vi "SQL_DB.vi"(3 "column information":T2[](array[typedef]), 4 "Column Names":T1=["Barcode", "[Date&Time]", "[User Name]", "Shift", "Model", "Variant", "[Test Name]", "[Test Type]", "[Excepted Value]", "HL", "LL", "[Obtained Value]", "Result", "[Cycle Time]"], 5 "datatype":string[][](array[string]), 6 "Table Name":string, 7 "CTRL":T4=enum."Open Connections", 8 "error in (no error)":errorcluster, 9 "SQL query":string, 10 "data to Update":variant, 11 "Connection Info":string="Provider=SQLNCLI11;Server=ADMIN-PC;Database=mmk;Trusted_Connection=yes;") -> (0 "error in (no error) 2":errorcluster, 1 "Data out 2":string[][](array[string]), 2 "Table/Columns":string[](array[string]))   [LabVIEW 2017]
uses:
  SQL_DB-Enum.ctl
  <vilib>/addons/database/Auxilliary.llb/DB Tools Column Info.ctl
  <vilib>/addons/database/Auxilliary.llb/DB Tools DataTypes.ctl
  Detailed Report/Controls/Detailed_Reports_Columns.ctl
  <vilib>/addons/database/Connection.llb/DB Tools Open Connec (String).vi
  <vilib>/addons/database/Connection.llb/Conn Execute.vi
  <vilib>/addons/database/Recordset.llb/Rec Fetch Recordset Data (R).vi
  <vilib>/addons/database/Recordset.llb/Rec Destroy - Connection.vi
  <vilib>/addons/database/_DB Variant To Data/Database Variant To Data.xnode
  <vilib>/addons/database/NI_Database_API.lvlib
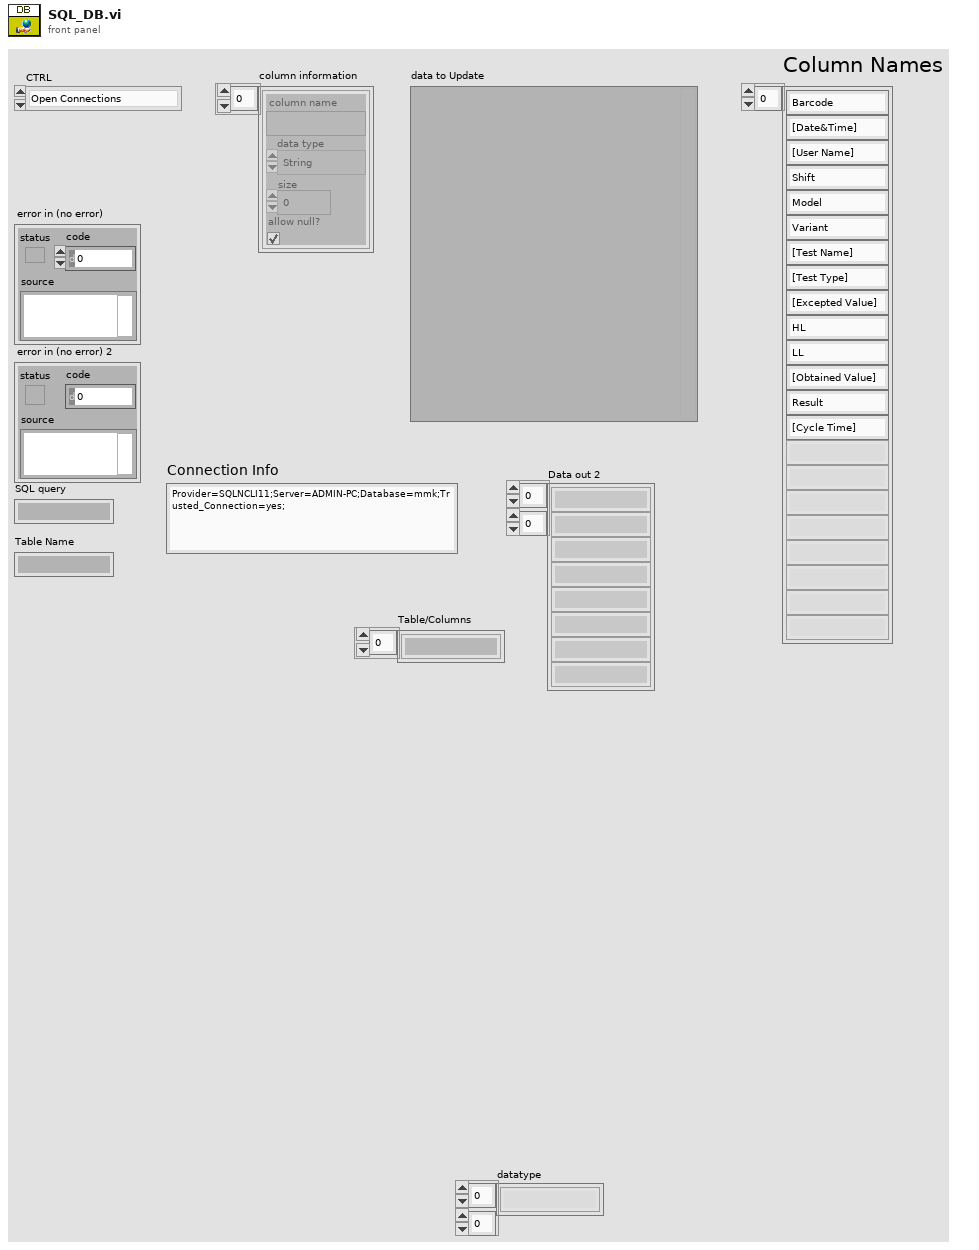
[diagram p1: front panel]
types:
  T1 = typedef "Detailed_Reports_Columns.ctl" = string[]
  T2 = typedef "NI_Database_API.lvlib/DB Tools Column Info.ctl" = cluster{"column name":string, "data type":T3, "size":i32, "allow null?":bool}
  T3 = typedef "NI_Database_API.lvlib/DB Tools DataTypes.ctl" = enum16{"String", "Long (I32)", "Single (SGL)", "Double (DBL)", "Date/Time", "Binary"}
  T4 = typedef "SQL_DB-Enum.ctl" = enum16{"INI DATA", "Open Connections", "Query", "Update Table", "Get Full Report", "Get Serial Numbers", "Get Table Columns", "Get Table Names", "Check & Create Table", "Close Connection"}
  T5 = typedef "NI_Database_API.lvlib/Conn ObjectReference.ctl" = refnum<k1>
  T6 = typedef "NI_Database_API.lvlib/Rec ObjectReference.ctl" = refnum<k1>
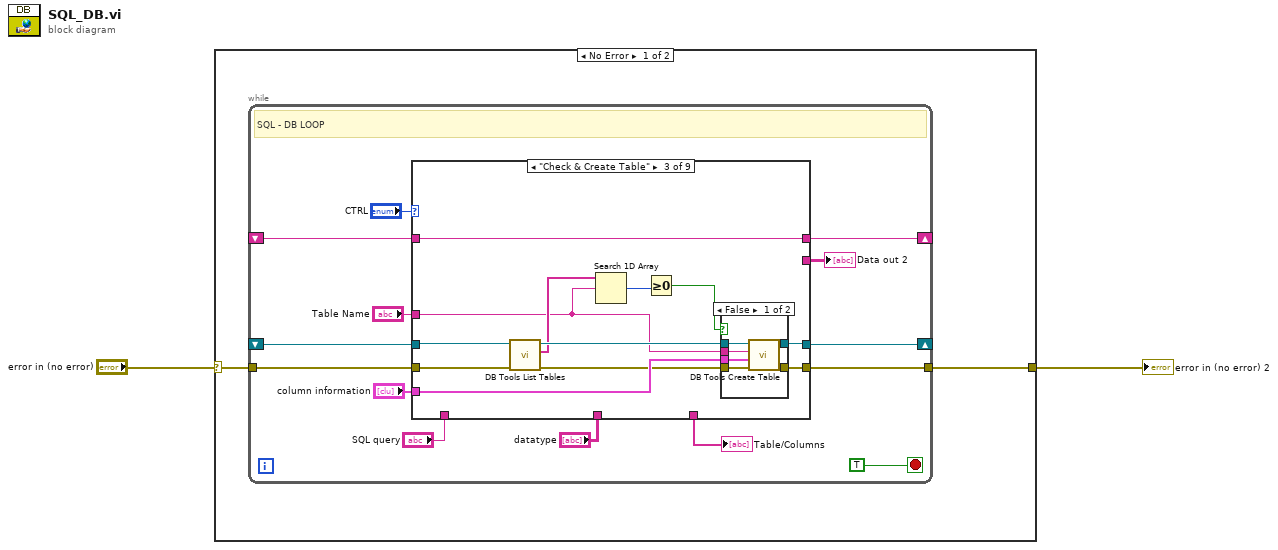
[diagram p0: block diagram]
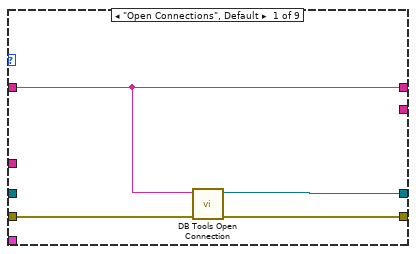
[diagram p2: hidden frame]
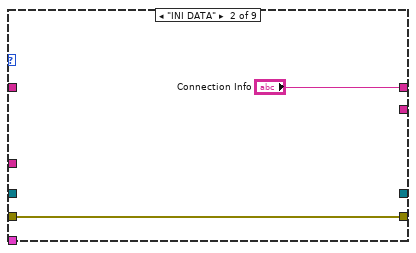
[diagram p3: hidden frame]
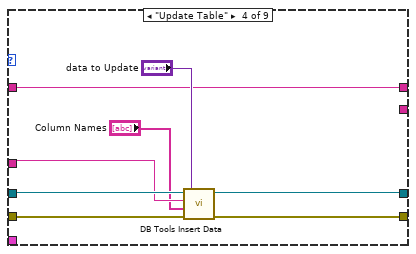
[diagram p5: hidden frame]
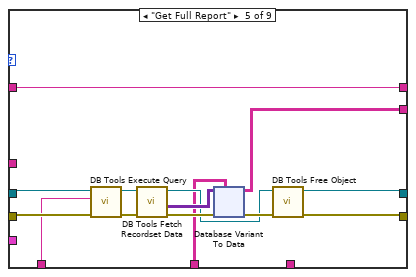
[diagram p6: hidden frame]
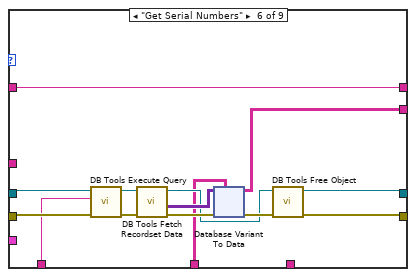
[diagram p7: hidden frame]
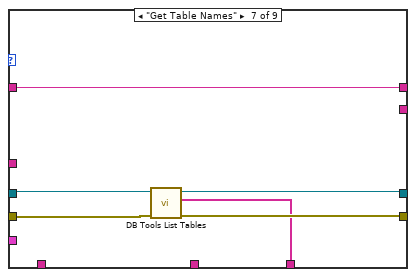
[diagram p8: hidden frame]
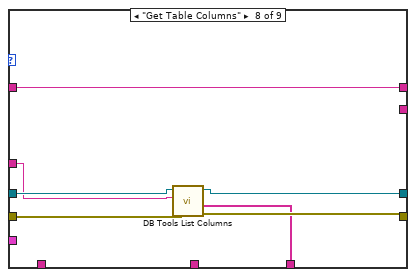
[diagram p9: hidden frame]
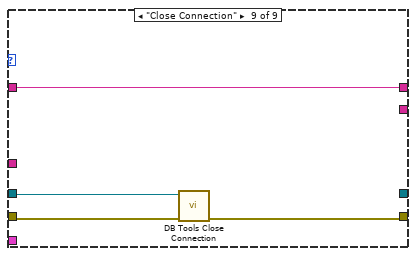
[diagram p10: hidden frame]
diagram:
  n1 = case shown="No Error" "error in (no error)" {
    selector: "error in (no error)" -> [w4 w186]
    tunnel: [w3 w186] -> w1
    frame No Error {
      n2 = while "SQL - DB LOOP" {
        tunnel: w4 -> [w17]
        tunnel: [w16] -> w3
        shift-right: [w15] -> _
        shift-left: _ -> [w14]
        shift-right: [w9] -> _
        shift-left: _ -> [w8]
        stop <- TRUE stop-if-true
        # "SQL - DB LOOP"
        n3 = case shown="\"Check & Create Table\"" "CTRL" {
          tunnel: w17 -> [w22 w23 w32 w52 w60 w118 w173 w179 w185]
          tunnel: [w21 w23 w36 w51 w59 w117 w171 w178 w184] -> w16
          tunnel: [w20 _ w35 w48 w58 w116 w170 w177 _] -> w15
          tunnel: w14 -> [_ _ w31 w50 w57 w115 w172 w180 w183]
          tunnel: "SQL query" -> [_ _ _ _ w56 w114 _ _ _]
          tunnel: "datatype" -> [_ _ _ _ w55 w113 _ _ _]
          tunnel: [_ _ _ _ w54 w112 _ _ _] -> w10
          tunnel: [w19 "Connection Info" w34 w47 w53 w111 w174 w181 w182] -> w9
          tunnel: w8 -> [w19 _ w34 w47 w53 w111 w174 w181 w182]
          tunnel: [_ _ _ _ _ _ w169 w176 _] -> w7
          tunnel: "Table Name" -> [_ _ w28 w46 _ _ _ w175 _]
          tunnel: "column information" -> [_ _ w33 _ _ _ _ _ _]
          frame "Open Connections", Default {
            n4 = call-poly <vilib>:"DB Tools Open Connection.vi"("error in (no error)"=w22, "connection information"=w19) -> ("error out"=w21:errorcluster, "connection reference"=w20:T5)  [unwired: 6 in]
          }
          frame "INI DATA" {
          }
          frame "Check & Create Table" {
            n5 = call <vilib>:"DB Tools List Tables.vi"("error in (no error)"=w32, "connection reference"=w31) -> ("error out"=w25:errorcluster, "tables"=w29:string[], "connection reference out"=w30:T5)  [unwired: 3 in]
            n6 = Search 1D Array(1D array=w29, element=w28) -> (index of element=w27:i32)  [unwired: 1 in]
            n7 = Greater Or Equal To 0?(x=w27) -> (x >= 0?=w26:bool)
            n8 = case shown="False" w26 {
              tunnel: [w42 w43] -> w36
              tunnel: [w41 w44] -> w35
              tunnel: w33 -> [w40 _]
              tunnel: w25 -> [w39 w43]
              tunnel: w30 -> [w38 w44]
              tunnel: w28 -> [w37 _]
              frame False {
                n9 = call <vilib>:"DB Tools Create Table.vi"("error in (no error)"=w39, "column information"=w40, "table"=w37, "connection reference"=w38) -> ("error out"=w42:errorcluster, "connection reference out"=w41:T5)  [unwired: 4 in]
              }
              frame True {
              }
            }
          }
          frame "Update Table" {
            n10 = call <vilib>:"DB Tools Insert Data.vi"("data"="data to Update", "error in (no error)"=w52, "columns"="Column Names", "table"=w46, "connection reference"=w50) -> ("error out"=w51:errorcluster, "connection reference out"=w48:T5)  [unwired: 5 in]
          }
          frame "Get Full Report" {
            n11 = call-poly <vilib>:"DB Tools Execute Query.vi"("error in (no error)"=w60, "SQL query"=w56, "connection reference"=w57) -> ("error out"=w66:errorcluster, "recordset reference"=w65:T6)  [unwired: 5 in]
            n12 = call-poly <vilib>:"DB Tools Fetch Recordset Data.vi"("error in (no error)"=w66, "recordset reference"=w65) -> ("error out"=w64:errorcluster, "recordset data"=w63:variant[][], "recordset reference out"=w61:T6)  [unwired: 3 in]
            n13 = xnode "Database Variant To Data"("database variant"=w63, "error in"=w64, "type"=w55) -> ("data"=w54:string[][], "error out"=w62:errorcluster)
            n14 = call-poly <vilib>:"DB Tools Free Object.vi"("error in (no error)"=w62, "recordset reference"=w61) -> ("error out"=w59:errorcluster, "connection reference"=w58:T5)  [unwired: 8 in]
          }
          frame "Get Serial Numbers" {
            n15 = call-poly <vilib>:"DB Tools Execute Query.vi"("error in (no error)"=w118, "SQL query"=w114, "connection reference"=w115) -> ("error out"=w124:errorcluster, "recordset reference"=w123:T6)  [unwired: 5 in]
            n16 = call-poly <vilib>:"DB Tools Fetch Recordset Data.vi"("error in (no error)"=w124, "recordset reference"=w123) -> ("error out"=w122:errorcluster, "recordset data"=w121:variant[][], "recordset reference out"=w119:T6)  [unwired: 3 in]
            n17 = xnode "Database Variant To Data"("database variant"=w121, "error in (no error)"=w122, "type"=w113) -> ("data"=w112:string[][], "error out"=w120:errorcluster)
            n18 = call-poly <vilib>:"DB Tools Free Object.vi"("error in (no error)"=w120, "recordset reference"=w119) -> ("error out"=w117:errorcluster, "connection reference"=w116:T5)  [unwired: 8 in]
          }
          frame "Get Table Names" {
            n19 = call <vilib>:"DB Tools List Tables.vi"("error in (no error)"=w173, "connection reference"=w172) -> ("error out"=w171:errorcluster, "tables"=w169:string[], "connection reference out"=w170:T5)  [unwired: 3 in]
          }
          frame "Get Table Columns" {
            n20 = call <vilib>:"DB Tools List Columns.vi"("error in (no error)"=w179, "table"=w175, "connection reference"=w180) -> ("error out"=w178:errorcluster, "columns"=w176:string[], "connection reference out"=w177:T5)  [unwired: 1 in, 1 out]
          }
          frame "Close Connection" {
            n21 = call <vilib>:"DB Tools Close Connection.vi"("error in (no error)"=w185, "connection reference"=w183) -> ("error out"=w184:errorcluster)  [unwired: 5 in]
          }
        }
        "Data out 2" <- w10
        "Table/Columns" <- w7
      }
    }
    frame Error {
    }
  }
  "error in (no error) 2" <- w1
